vi "GenerateScreenShots.vi"() -> ()   [LabVIEW 2012]
panel:
  out "Modified VIs":path[](array[path])
  out "Number of VI found":i32
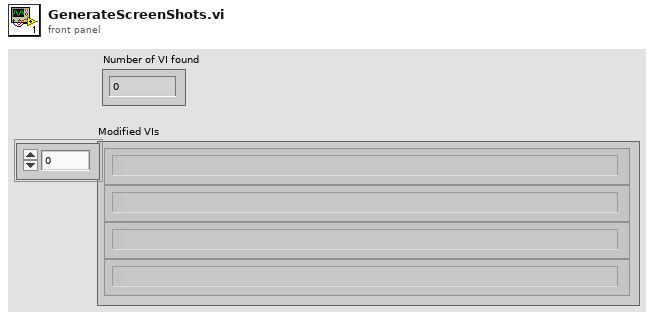
[diagram p1: front panel]
types:
  T1 = cluster{"result string":string, "result string":string}
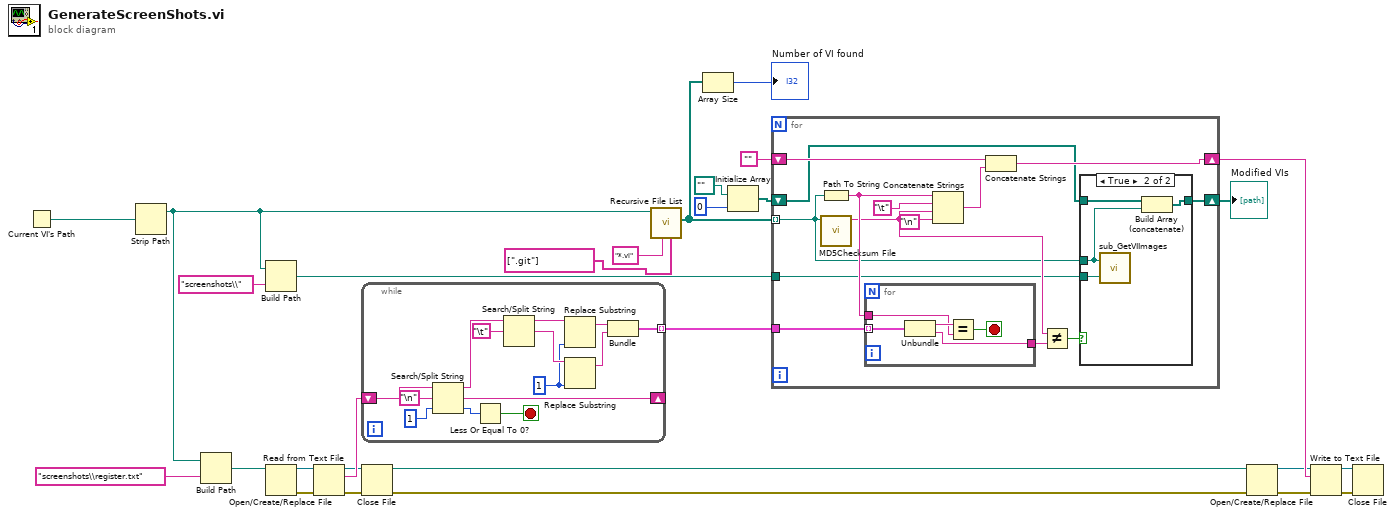
[diagram p0: block diagram]
diagram:
  n1 = Current VI's Path() -> (path=w26:path)
  n2 = Strip Path(path=w26) -> (stripped path=w6:path)  [unwired: 1 out]
  n3 = Build Path(base path=w6, name or relative path="screenshots\\register.txt") -> (appended path=w20:path)
  n4 = Build Path(base path=w6, name or relative path="screenshots\\") -> (appended path=w8:path)
  n5 = Open/Create/Replace File(file path (use dialog)=w20) -> (refnum out=w19:refnum<file>, error out=w18:errorcluster)  [unwired: 5 in, 1 out]
  n6 = Read from Text File(file (use dialog)=w19, error in=w18) -> (refnum out=w16:refnum<file>, text=w21:string, error out=w17:errorcluster)  [unwired: 2 in, 1 out]
  n7 = while {
    tunnel: [w37] -> w9 mode=indexing
    shift-right: [w32] -> _
    shift-left: w21 -> [w42]
    stop <- w41 stop-if-true
    w29 = 1 ("offset (0)")
    n8 = Search/Split String(string=w42, search string/char (-)="\n", offset (0)=1) -> (substring before match=w38:string, match + rest of string=w32:string, offset of match=w40:i32)
    n9 = Less Or Equal To 0?(x=w40) -> (x <= 0?=w41:bool)
    n10 = Search/Split String(string=w38, search string/char (-)="\t") -> (substring before match=w30:string, match + rest of string=w35:string)  [unwired: 1 in, 1 out]
    n11 = Replace Substring(2:w29, 5:w30) -> (1:w31:string)  [unwired: 2 in, 1 out]
    n12 = Replace Substring(2:w29, 5:w35) -> (1:w36:string)  [unwired: 2 in, 1 out]
    n13 = Bundle("result string"=w31, "result string"=w36) -> (w37:T1)  [unwired: 1 in]
  }
  n14 = Close File(refnum=w16, error in=w17) -> (path=w11:path, error out=w10:errorcluster)
  n15 = call <vilib>:"Recursive File List.vi"("Folders to Exclude"=string[] [".git"], "pattern"="*.vi", "Folder Path"=w6) -> ("All Files in Dir"=w23:path[])  [unwired: 4 in, 4 out]
  n16 = Array Size(array=w23) -> (size(s)=→"Number of VI found":i32)
  n17 = Initialize Array(path "", 0 ("dimension size")) -> (w4:path[])
  n18 = for {
    tunnel: w23 -> [w51] mode=indexing
    tunnel: w9 -> [w49]
    tunnel: w8 -> [w50]
    shift-right: [w46] -> w22
    shift-left: "" -> [w48]
    shift-right: [w44] -> w1
    shift-left: w4 -> [w43]
    n19 = Path To String(path=w51) -> (string=w55:string)
    n20 = call <vilib>:"MD5Checksum File.vi"("Path"=w51) -> ("MD5 message-digest"=w53:string)  [unwired: 9 in, 1 out]
    n21 = for {
      tunnel: w55 -> [w65]
      tunnel: [w63] -> w54
      tunnel: w49 -> [w62] mode=indexing
      stop <- w64 stop-if-true
      n22 = Unbundle(w62) -> ("result string"=w66:string, "result string"=w63:string)
      n23 = Equal?(x=w66, y=w65) -> (x = y?=w64:bool)
    }
    n24 = Concatenate Strings(w55, "\t", w53, "\n") -> (w47:string)
    n25 = Concatenate Strings(w48, w47) -> (w46:string)
    n26 = Not Equal?(x=w53, y=w54) -> (x != y?=w52:bool)
    n27 = case shown="True" w52 {
      tunnel: w51 -> [_ w58]
      tunnel: w50 -> [_ w61]
      tunnel: w43 -> [w57 w60]
      tunnel: [w57 w59] -> w44
      frame False {
      }
      frame True {
        n28 = call "sub_GetVIImages.vi"("Save screenshot dir"=w61, "Selected VI"=w58) -> ()  [unwired: 2 out]
        n29 = Build Array (concatenate)(w60, w58) -> (w59:path[])
      }
    }
  }
  "Modified VIs" <- w1
  n30 = Open/Create/Replace File(file path (use dialog)=w11, error in=w10) -> (refnum out=w14:refnum<file>, error out=w15:errorcluster)  [unwired: 4 in, 1 out]
  n31 = Write to Text File(file (use dialog)=w14, text=w22, error in=w15) -> (refnum out=w13:refnum<file>, error out=w12:errorcluster)  [unwired: 1 in, 1 out]
  n32 = Close File(refnum=w13, error in=w12) -> ()  [unwired: 2 out]
